vi "Set value_MFP3D.vi"(9 "Number resolutio":string="%.7f)", 10 "Value":dbl=0.1 format="%_5p", 11 "Output":u16(ring) items=["OutA_52kHz", "OutB_52kHz", "OutC_78Hz", "PiezoX", "PiezoY", "PiezoZ", "DDS_Frequency1", "DDS_Frequency2", "DDS_Amplitude1", "DDS_Amplitude2", "DDS_DCOffset", "\"Setpoint%PIDSLoop.3\"", "\"Setpoint%PIDSLoop.4\"", ""]) -> (3 "error out":errorcluster={"status"=FALSE, "code"=0, "source"="DDE Request: No Error"})   [LabVIEW 2019]
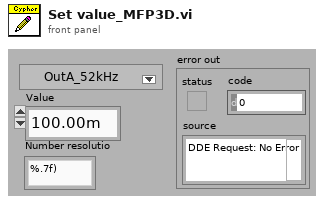
[diagram p1: front panel]
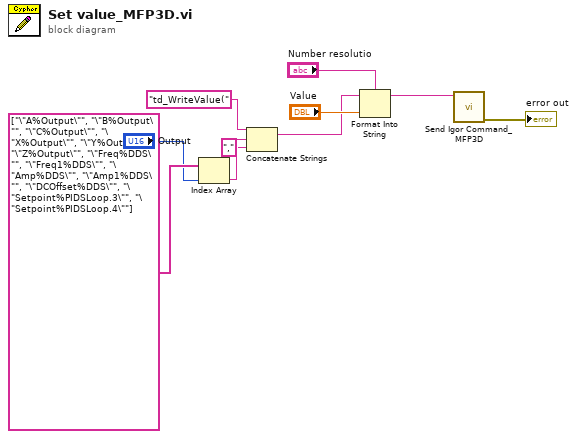
[diagram p0: block diagram]
diagram:
  n1 = Index Array(array=string[] ["\"A%Output\"", "\"B%Output\"", "\"C%Output\"", "\"X%Output\"", "\"Y%Output\"", "\"Z%Output\"", "\"Freq%DDS\"", "\"Freq1%DDS\"", "\"Amp%DDS\"", "\"Amp1%DDS\"", "\"DCOffset%DDS\"", "\"Setpoint%PIDSLoop.3\"", "\"Setpoint%PIDSLoop.4\""], index="Output") -> (element=w5:string)
  n2 = Concatenate Strings("td_WriteValue(", w5, "," ("string")) -> (w4:string)
  n3 = Format Into String "Format Into String"(format string="Number resolutio", initial string=w4, "Value") -> (resulting string=w2:string)  [unwired: 1 in, 1 out]
  n4 = call "Send Igor Command_MFP3D.vi"("Command"=w2) -> ("error out"=→"error out":errorcluster)  [unwired: 7 in, 2 out]
